vi "Lidar Distance Global.vi"() -> ()   [LabVIEW 2014]
panel:
  in  "Lidar_Distance":dbl
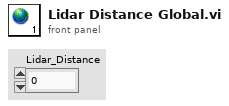
[diagram p1: front panel]
diagram:
